vi "Are Colliding.vi"(3 "Other Object in":refnum<class "SimulationObject.lvclass">, 5 "Self Object in":refnum<class "SimulationObject.lvclass">) -> (0 "Other Object out":refnum<class "SimulationObject.lvclass">, 1 "Are Colliding":bool, 2 "Self Object out":refnum<class "SimulationObject.lvclass">)   [LabVIEW 2022 SP3, in "Collider.lvclass"]
uses:
  Collider.lvclass
  SimulationObject/SimulationObject.lvclass
  Circle Collider/Circle Collider.lvclass
  SimulationObject/SimulationObject.lvclass/SimulationObject.ctl
  Rect Collider/Rect Collider.lvclass
  Collider.lvclass/Collider.ctl
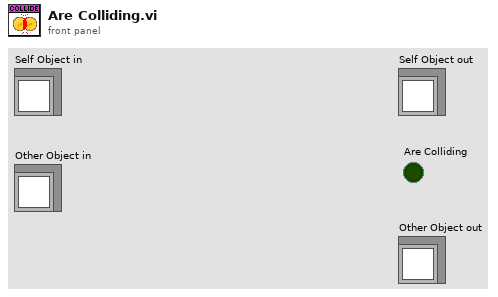
[diagram p1: front panel]
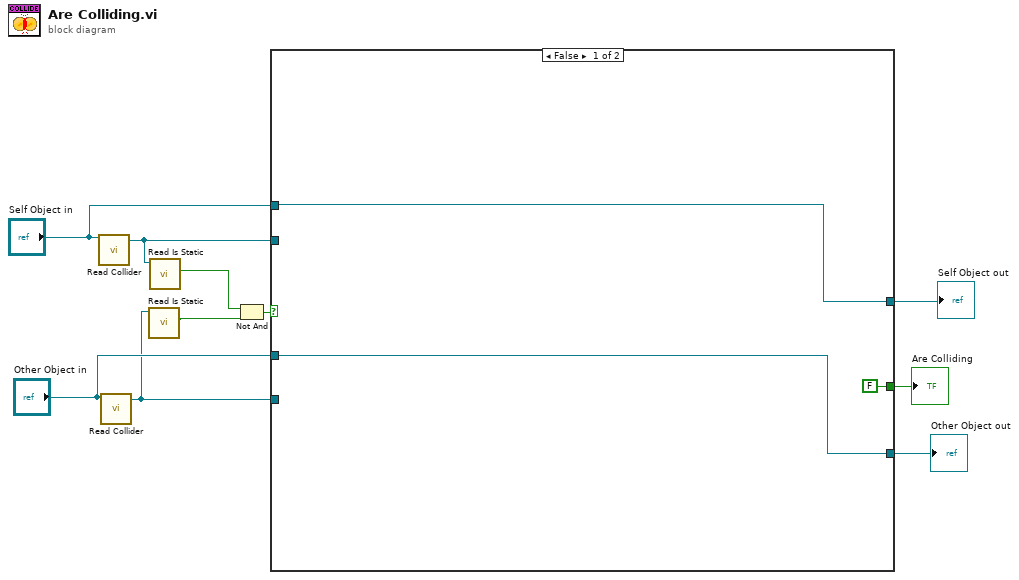
[diagram p0: block diagram]
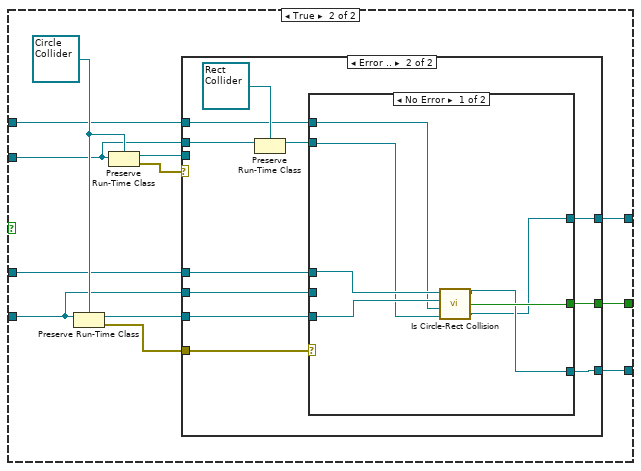
[diagram p2: hidden frame]
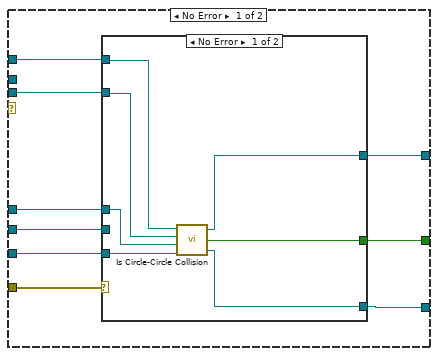
[diagram p3: hidden frame]
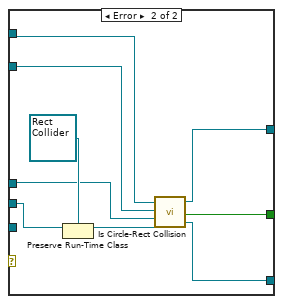
[diagram p4: hidden frame]
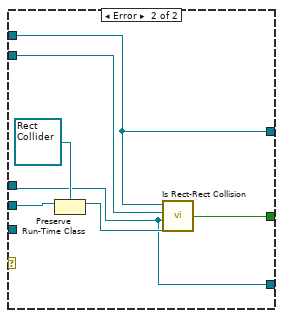
[diagram p5: hidden frame]
diagram:
  n1 = call "Read Collider.vi"("SimulationObject in"="Self Object in") -> ("Collider out"=w5:refnum<class "Collider.lvclass">)  [unwired: 8 in, 2 out]
  n2 = call "Read Collider.vi"("SimulationObject in"="Other Object in") -> ("Collider out"=w4:refnum<class "Collider.lvclass">)  [unwired: 8 in, 2 out]
  n3 = call "Read Is Static.vi"("Collider in"=w4) -> ("Is Static"=w1:bool)  [unwired: 8 in, 2 out]
  n4 = call "Read Is Static.vi"("Collider in"=w5) -> ("Is Static"=w2:bool)  [unwired: 8 in, 2 out]
  n5 = Not And(1:w1, 2:w2) -> (0:w3:bool)
  n6 = case shown="False" w3 {
    tunnel: w5 -> [_ w22]
    tunnel: w4 -> [_ w21]
    tunnel: "Self Object in" -> [w13 w18]
    tunnel: "Other Object in" -> [w12 w17]
    tunnel: [FALSE ("Are Colliding") w16] -> w8
    tunnel: [w13 w15] -> w7
    tunnel: [w12 w14] -> w6
    frame False {
    }
    frame True {
      w25 = refnum<class "Circle Collider.lvclass"> refnum ("Circle Collider.lvclass")
      n7 = Preserve Run-Time Class(object in=w21, 2:w25) -> (object out=w20:refnum<class "Circle Collider.lvclass">, error out=w19:errorcluster)  [unwired: 1 in]
      n8 = Preserve Run-Time Class(object in=w22, 2:w25) -> (object out=w23:refnum<class "Circle Collider.lvclass">, error out=w24:errorcluster)  [unwired: 1 in]
      n9 = case shown="Error .." w24 {
        tunnel: w23 -> [w32 _]
        tunnel: w22 -> [_ w61]
        tunnel: w21 -> [w28 w58]
        tunnel: w20 -> [w33 w53]
        tunnel: w19 -> [w34 w59]
        tunnel: w18 -> [w31 w55]
        tunnel: w17 -> [w30 w56]
        tunnel: [w29 w54] -> w16
        tunnel: [w27 w52] -> w15
        tunnel: [w26 w51] -> w14
        frame No Error {
          n10 = case shown="No Error" w34 {
            tunnel: w33 -> [w41 _]
            tunnel: w32 -> [w39 w47]
            tunnel: w31 -> [w38 w48]
            tunnel: w30 -> [w40 w46]
            tunnel: [w37 w44] -> w29
            tunnel: w28 -> [_ w49]
            tunnel: [w36 w43] -> w27
            tunnel: [w35 w42] -> w26
            frame No Error {
              n11 = call "Is Circle-Circle Collision.vi"("Other Collider"=w41, "Other object in"=w40, "Self Collider in"=w39, "Self Object in"=w38) -> ("Other Object out"=w35:refnum<class "SimulationObject.lvclass">, "Are Colliding"=w37:bool, "Self Object out"=w36:refnum<class "SimulationObject.lvclass">)
            }
            frame Error {
              n12 = Preserve Run-Time Class(object in=w49, 2:refnum<class "Rect Collider.lvclass"> refnum ("Rect Collider.lvclass")) -> (object out=w45:refnum<class "Rect Collider.lvclass">)  [unwired: 1 in, 1 out]
              n13 = call "Is Circle-Rect Collision.vi"("Other Collider in"=w45, "Other Object in"=w46, "Self Collider in"=w47, "Self Object in"=w48) -> ("Other Object out"=w42:refnum<class "SimulationObject.lvclass">, "Are Colliding"=w44:bool, "Self Object out"=w43:refnum<class "SimulationObject.lvclass">)
            }
          }
        }
        frame Error {
          n14 = Preserve Run-Time Class(object in=w61, 2:refnum<class "Rect Collider.lvclass"> refnum ("Rect Collider.lvclass")) -> (object out=w57:refnum<class "Rect Collider.lvclass">)  [unwired: 1 in, 1 out]
          n15 = case shown="No Error" w59 {
            tunnel: w58 -> [_ w74]
            tunnel: w57 -> [w65 w71]
            tunnel: w56 -> [w67 w69]
            tunnel: w55 -> [w64 w70]
            tunnel: [w68 w73] -> w54
            tunnel: w53 -> [w66 _]
            tunnel: [w62 w70] -> w52
            tunnel: [w63 w69] -> w51
            frame No Error {
              n16 = call "Is Circle-Rect Collision.vi"("Other Collider in"=w65, "Other Object in"=w64, "Self Collider in"=w66, "Self Object in"=w67) -> ("Other Object out"=w62:refnum<class "SimulationObject.lvclass">, "Are Colliding"=w68:bool, "Self Object out"=w63:refnum<class "SimulationObject.lvclass">)
            }
            frame Error {
              n17 = Preserve Run-Time Class(object in=w74, 2:refnum<class "Rect Collider.lvclass"> refnum ("Rect Collider.lvclass")) -> (object out=w72:refnum<class "Rect Collider.lvclass">)  [unwired: 1 in, 1 out]
              n18 = call "Is Rect-Rect Collision.vi"("Other Collider in"=w72, "Other object in"=w69, "Self Collider in"=w71, "Self Object in"=w70) -> ("Are Colliding"=w73:bool)
            }
          }
        }
      }
    }
  }
  "Are Colliding" <- w8
  "Self Object out" <- w7
  "Other Object out" <- w6
